vi "envio_labview_to_unity.vi"() -> ()   [LabVIEW 2017]
panel:
  in  "Stop 2":bool
  out "posicao_motores":dbl[](array[numeric])
  out "text":string
  in  "Stop":bool
  out "concatenated string":string
  out "Numeric Control":i32
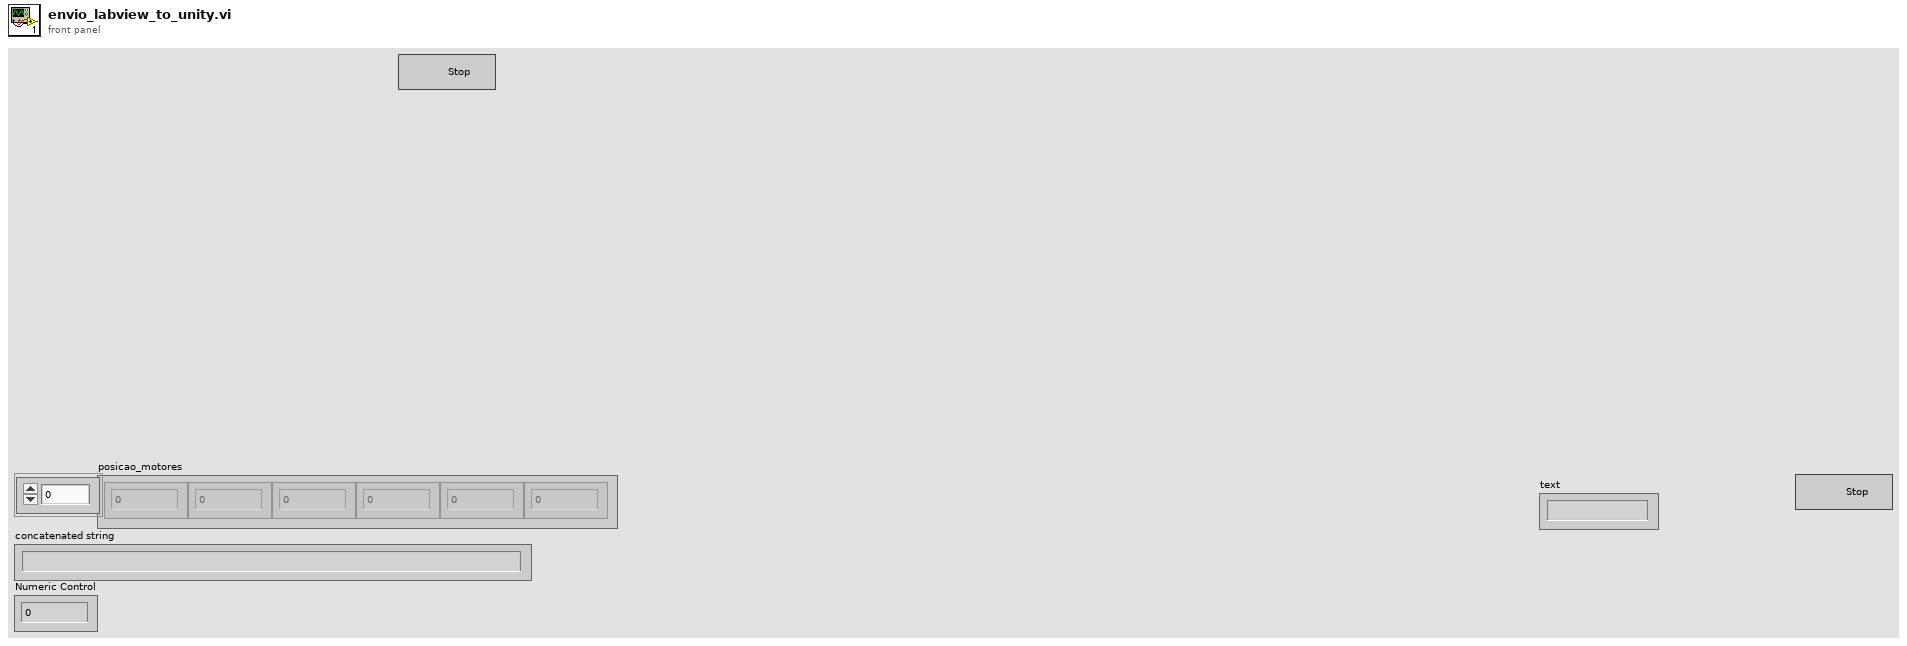
[diagram p1: front panel]
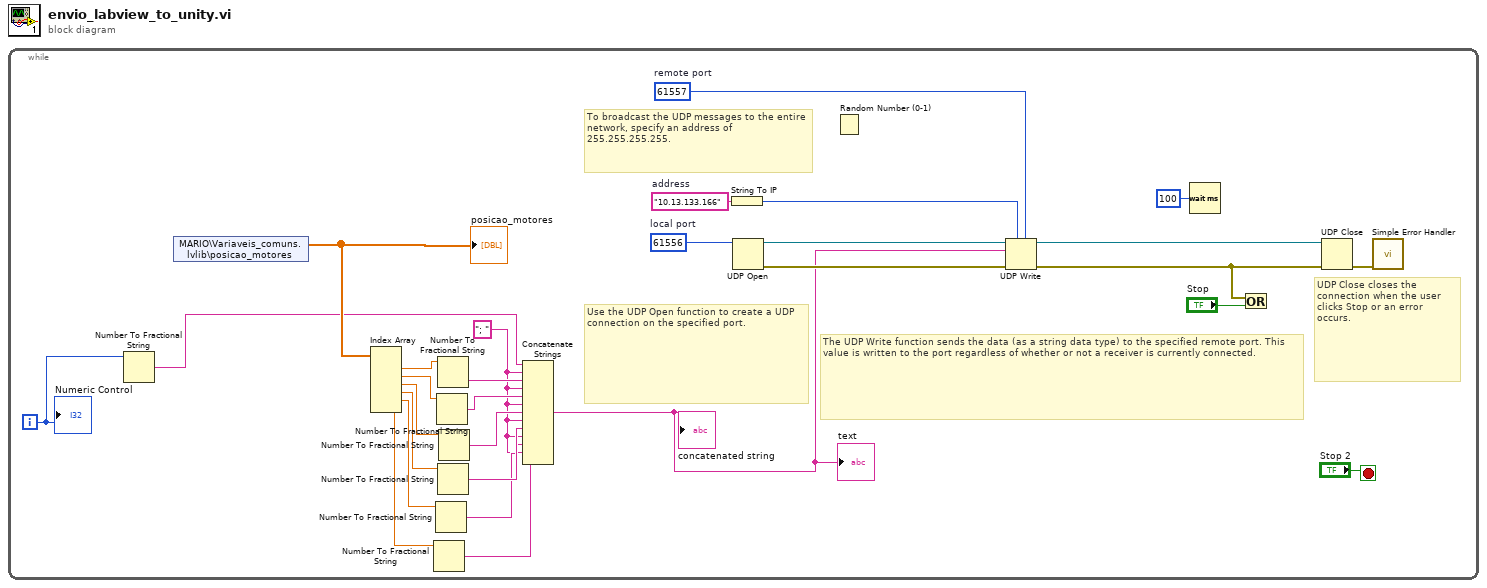
[diagram p0: block diagram]
diagram:
  n1 = while {
    i -> [w2]
    stop <- "Stop 2" stop-if-true
    w3 = "; " ("string")
    w20 = u16 61557  # remote port
    w21 = u16 61556  # local port
    w26 = "10.13.133.166"  # address
    # "To broadcast the UDP messages to the entire network, specify an address of 255.255.255.255."
    # "UDP Close closes the connection when the user clicks Stop or an error occurs."
    # "The UDP Write function sends the data (as a string data type) to the specified remote port. This value is written to the port regardless of whether or not a receiver is currently connected."
    # "Use the UDP Open function to create a UDP connection on the specified port."
    n2 = Number To Fractional String(number=w2) -> (F-format string=w1:string)  [unwired: 3 in]
    n3 = shared-variable "MARIO\\Variaveis_comuns.lvlib\\posicao_motores"() -> (w17:dbl[])  [unwired: 1 in, 1 out]
    "posicao_motores" <- w17
    n4 = Index Array(array=w17) -> (element #1=w16:dbl, element #2=w15:dbl, element #3=w14:dbl, element #4=w13:dbl, element #5=w12:dbl, element #6=w11:dbl)  [unwired: 6 in]
    n5 = Number To Fractional String(number=w11) -> (F-format string=w5:string)  [unwired: 3 in]
    n6 = Number To Fractional String(number=w12) -> (F-format string=w6:string)  [unwired: 3 in]
    n7 = Number To Fractional String(number=w15) -> (F-format string=w9:string)  [unwired: 3 in]
    n8 = Number To Fractional String(number=w16) -> (F-format string=w10:string)  [unwired: 3 in]
    n9 = Number To Fractional String(number=w13) -> (F-format string=w7:string)  [unwired: 3 in]
    n10 = Number To Fractional String(number=w14) -> (F-format string=w8:string)  [unwired: 3 in]
    n11 = Concatenate Strings(w1, w3, w10, w3, w9, w3, w8, w3, w7, w3, w6, w3, w5) -> (w4:string)
    "text" <- w4
    "concatenated string" <- w4
    n12 = String To IP(1:w26) -> (0:w24:u32)
    n13 = UDP Open(11:w21) -> (port=w23:refnum<k16>, 0:w22:errorcluster)  [unwired: 4 in, 1 out]
    n14 = Random Number (0-1)() -> ()  [unwired: 1 out]
    n15 = UDP Write(address=w24, port or service name=w20, connection ID=w23, data in=w4, 8:w22) -> (error out=w27:errorcluster, 3:w28:refnum<k16>)  [unwired: 1 in]
    n16 = Wait (ms)(milliseconds to wait=u32 100) -> ()  [unwired: 1 out]
    n17 = Or(x=w27, y="Stop") -> ()  [unwired: 1 out]
    n18 = UDP Close(connection ID=w28, 8:w27) -> (error out=w25:errorcluster)  [unwired: 1 out]
    n19 = call <vilib>:"Simple Error Handler.vi"("error in (no error)"=w25) -> ()  [unwired: 4 in, 5 out]
    "Numeric Control" <- w2
  }
